vi "__init__.vi"(8 "error in (no error)":errorcluster, 11 "self in":refnum<class "SymbolRefId.lvclass">) -> (0 "error out":errorcluster, 3 "self out":refnum<class "SymbolRefId.lvclass">)   [LabVIEW 2020, in "mlir.lvlib" / "SymbolRefId.lvclass"]
uses:
  SymbolRefId.lvclass
  SymbolRefId.lvclass/SymbolRefId.ctl
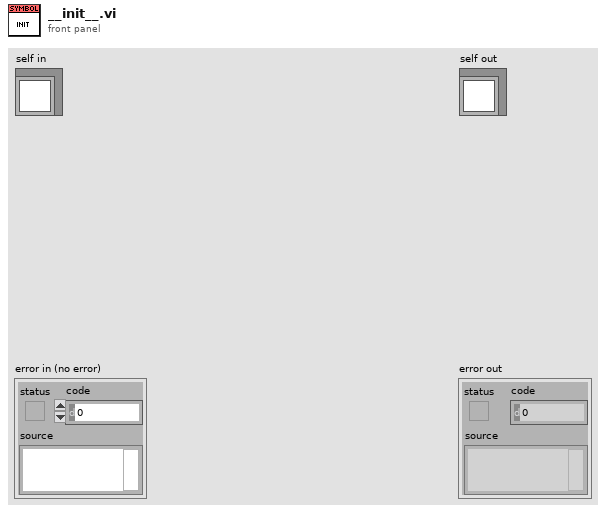
[diagram p1: front panel]
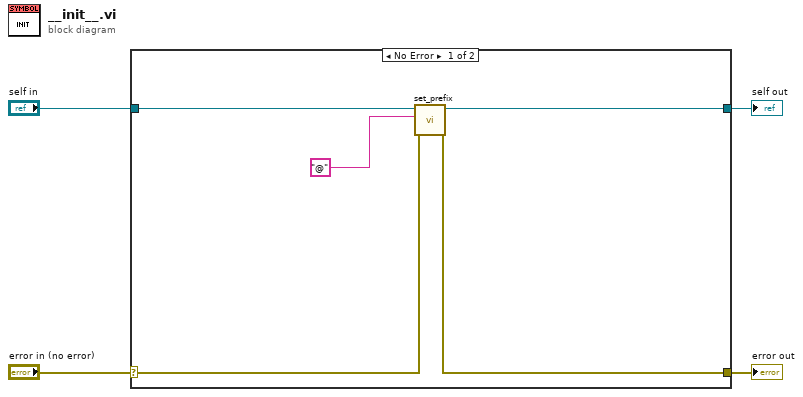
[diagram p0: block diagram]
diagram:
  n1 = case shown="No Error" "error in (no error)" {
    selector: "error in (no error)" -> [w6 w11]
    tunnel: [w5 w11] -> w3
    tunnel: [w8 w10] -> w1
    tunnel: "self in" -> [w9 w10]
    frame No Error {
      n2 = call-dynamic "set_prefix.vi"("error in (no error)"=w6, "_prefix_"="@", "Identifier in"=w9) -> ("error out"=w5:errorcluster, "Identifier out"=w8:refnum<class "SymbolRefId.lvclass">)  [unwired: 7 in]
    }
    frame Error {
    }
  }
  "error out" <- w3
  "self out" <- w1
